vi "DELETE FROM DB.vi"(8 "error in (no error)":errorcluster, 10 "object":refnum<class "_ISerializable.lvclass">, 11 "orm in":refnum<class "LV-ORM.lvclass">) -> (0 "error out":errorcluster, 3 "orm out":refnum<class "LV-ORM.lvclass">)   [LabVIEW 2018, in "LV-ORM.lvclass"]
uses:
  LV-ORM.lvclass
  _Serializable Base Object/_ISerializable.lvclass
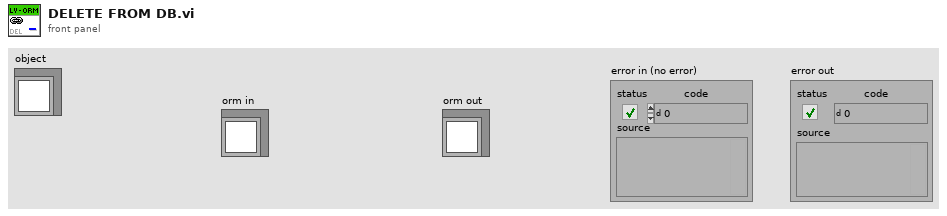
[diagram p1: front panel]
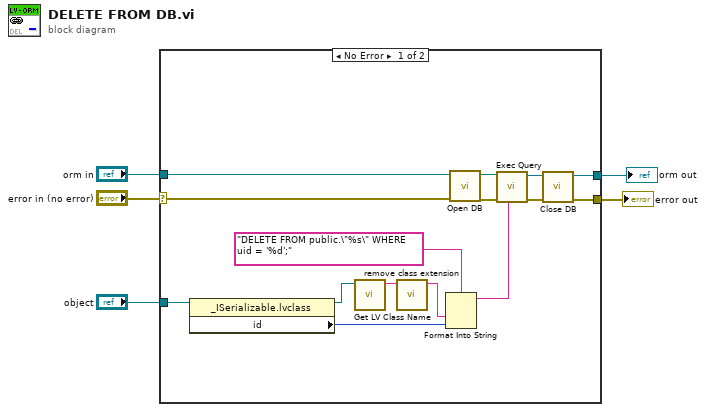
[diagram p0: block diagram]
diagram:
  n1 = case shown="No Error" "error in (no error)" {
    selector: "error in (no error)" -> [w14 w22]
    tunnel: "orm in" -> [w15 w21]
    tunnel: [w13 w22] -> w3
    tunnel: [w12 w21] -> w2
    tunnel: "object" -> [w6 _]
    frame No Error {
      n2 = property class="_ISerializable.lvclass"(reference=w6) -> (reference out=w18:refnum<class "_ISerializable.lvclass">, "id"=w17:i32)  [unwired: 1 in, 1 out]
      n3 = call <vilib>:"Get LV Class Name.vi"("object"=w18) -> ("class name"=w19:string)  [unwired: 9 in, 1 out]
      n4 = call "remove class extension.vi"("class name in"=w19) -> ("class name out"=w16:string)  [unwired: 10 in]
      n5 = Format Into String(format string="DELETE FROM public.\"%s\" WHERE uid = '%d';", w16, w17) -> (resulting string=w7:string)  [unwired: 2 in, 1 out]
      n6 = call "Open DB.vi"("error in (no error)"=w14, "LV-ORM in"=w15) -> ("error out"=w9:errorcluster, "LV-ORM out"=w8:refnum<class "LV-ORM.lvclass">)  [unwired: 8 in]
      n7 = call "Exec Query.vi"("scripts"=w7, "error in"=w9, "orm in"=w8) -> ("error out"=w10:errorcluster, "orm out"=w11:refnum<class "LV-ORM.lvclass">)  [unwired: 7 in]
      n8 = call "Close DB.vi"("error in"=w10, "LV-ORM in"=w11) -> ("error out"=w13:errorcluster, "LV-ORM out"=w12:refnum<class "LV-ORM.lvclass">)  [unwired: 8 in]
    }
    frame Error {
    }
  }
  "orm out" <- w2
  "error out" <- w3
